vi "OP60 Indicators.vi"(8 "error in (no error)":errorcluster, 10 "Array":refnum<vi>[](array[refnum]), 11 "OUTPUT INDICATOR in":T1) -> (0 "error out":errorcluster, 3 "OUTPUT INDICATOR out":T1)   [LabVIEW 2017]
uses:
  c1426024-f760-4962-9ceb-df5698c3b79e.vi
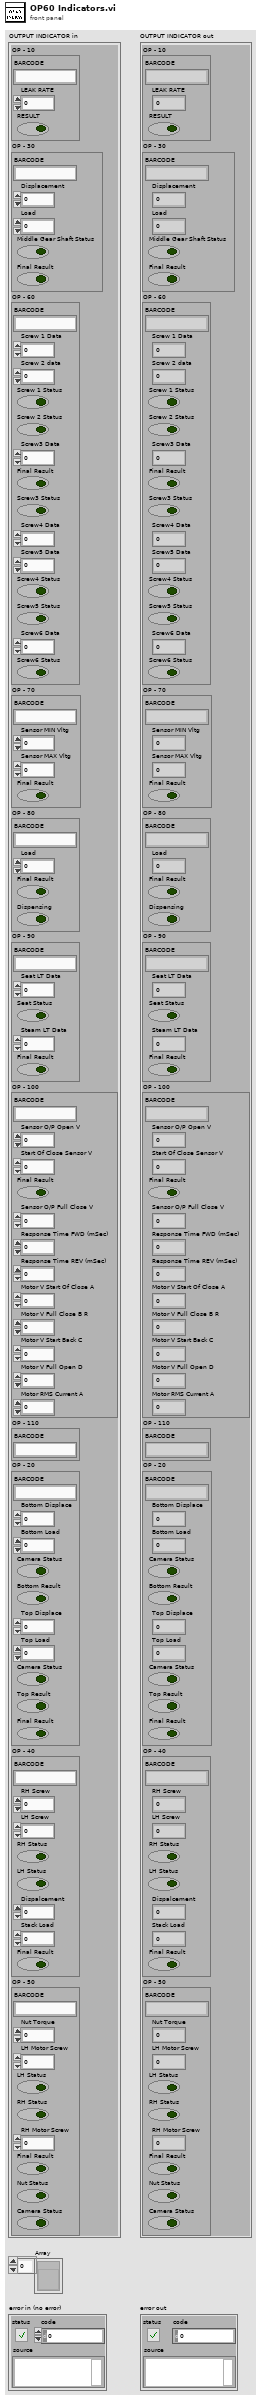
[diagram p1: front panel]
types:
  T1 = cluster{"OP - 10":cluster{"BARCODE":string, "LEAK RATE":dbl, "RESULT":bool}, "OP - 30":cluster{"BARCODE":string, "Displacement":dbl, "Load":dbl, "Middle Gear Shaft Status":bool, "Final Result":bool}, "OP - 60":cluster{"BARCODE":string, "Screw 1 Data":dbl, "Screw 2 data":dbl, "Screw 1 Status":bool, "Screw 2 Status":bool, "Screw3 Data":dbl, "Final Result":bool, "Screw3 Status":bool, "Screw4 Data":dbl, "Screw5 Data":dbl, "Screw4 Status":bool, "Screw5 Status":bool, "Screw6 Data":dbl, "Screw6 Status":bool}, "OP - 70":cluster{"BARCODE":string, "Sensor MIN Vltg":dbl, "Sensor MAX Vltg":dbl, "Final Result":bool}, "OP - 80":cluster{"BARCODE":string, "Load":dbl, "Final Result":bool, "Dispensing":bool}, "OP - 90":cluster{"BARCODE":string, "Seat LT Data":dbl, "Seat Status":bool, "Steam LT Data":dbl, "Final Result":bool}, "OP - 100":cluster{"BARCODE":string, "Sensor O/P Open V":dbl, "Start Of Close Sensor V":dbl, "Final Result":bool, "Sensor O/P Full Close V":dbl, "Response Time FWD (mSec)":dbl, "Response Time REV (mSec)":dbl, "Motor V Start Of Close A":dbl, "Motor V Full Close B R":dbl, "Motor V Start Back C":dbl, "Motor V Full Open D":dbl, "Motor RMS Current A":dbl}, "OP - 110":cluster{"BARCODE":string}, "OP - 20":cluster{"BARCODE":string, "Bottom Displace":dbl, "Bottom Load":dbl, "Camera Status":bool, "Bottom Result":bool, "Top Displace":dbl, "Top Load ":dbl, "Camera Status":bool, "Top Result":bool, "Final Result":bool}, "OP - 40":cluster{"BARCODE":string, "RH Screw":dbl, "LH Screw ":dbl, "RH Status":bool, "LH Status":bool, "Dispalcement ":dbl, "Stack Load ":dbl, "Final Result":bool}, "OP - 50":cluster{"BARCODE":string, "Nut Torque":dbl, "LH Motor Screw":dbl, "LH Status":bool, "RH Status":bool, "RH Motor Screw":dbl, "Final Result":bool, "Nut Status":bool, "Camera Status":bool}}
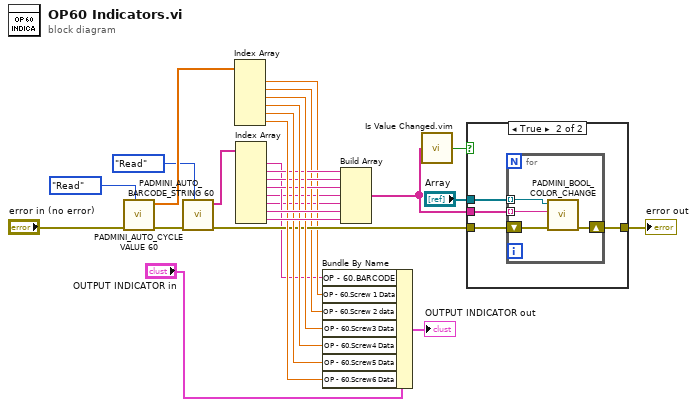
[diagram p0: block diagram]
diagram:
  n1 = call "PADMINI_AUTO_CYCLE VALUE 60.vi"("Enum"=enum16{"Read", "Write"}."Read", "error in (no error)"="error in (no error)") -> ("error out"=w13:errorcluster, "Input 2"=w17:sgl[])  [unwired: 8 in]
  n2 = call "PADMINI_AUTO_BARCODE_STRING 60.vi"("Enum"=enum16{"Read", "Write"}."Read", "error in (no error)"=w13) -> ("error out"=w15:errorcluster, "Input 2"=w16:string[])  [unwired: 8 in]
  n3 = Index Array(array=w17) -> (element #1=w5:sgl, element #2=w4:sgl, element #3=w20:sgl, element #4=w21:sgl, element #5=w22:sgl, element #6=w23:sgl)  [unwired: 6 in]
  n4 = Index Array(array=w16) -> (element #1=w3:string, element #2=w7:string, element #3=w8:string, element #4=w10:string, element #5=w2:string, element #6=w1:string, element #7=w24:string, element #8=w25:string)  [unwired: 8 in]
  n5 = Bundle By Name(cluster="OUTPUT INDICATOR in", "OP - 60.BARCODE"=w3, "OP - 60.Screw 1 Data"=w5, "OP - 60.Screw 2 data"=w4, "OP - 60.Screw3 Data"=w20, "OP - 60.Screw4 Data"=w21, "OP - 60.Screw5 Data"=w22, "OP - 60.Screw6 Data"=w23) -> (→"OUTPUT INDICATOR out":T1)
  n6 = Build Array(w7, w8, w10, w2, w1, w24, w25) -> (w9:string[])
  n7 = call "Is Value Changed.vim"("value"=w9) -> ("changed or first call?"=w6:bool)
  n8 = case shown="True" w6 {
    tunnel: [w28 w32] -> w26
    tunnel: w9 -> [_ w31]
    tunnel: w15 -> [w28 w30]
    tunnel: "Array" -> [_ w29]
    frame False {
    }
    frame True {
      n9 = for {
        tunnel: w31 -> [w35] mode=indexing
        shift-right: [w36] -> w32
        shift-left: w30 -> [w34]
        tunnel: w29 -> [w33] mode=indexing
        n10 = call "PADMINI_BOOL_COLOR_CHANGE.vi"("error in (no error)"=w34, "Input Result"=w35, "Boolean in"=w33) -> ("error out"=w36:errorcluster)  [unwired: 8 in]
      }
    }
  }
  "error out" <- w26
